vi "flame.vi"() -> ()   [LabVIEW 2017]
panel:
  in  "?":bool
  out "?":u16(ring)
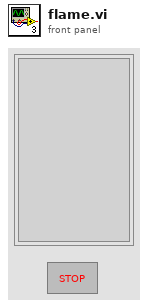
[diagram p1: front panel]
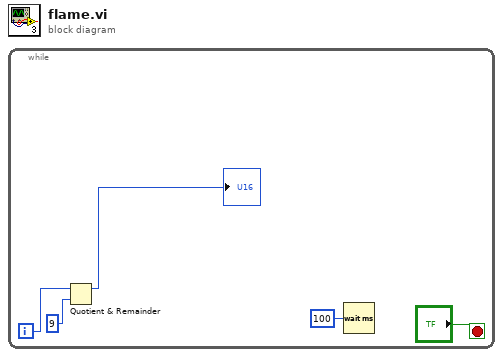
[diagram p0: block diagram]
diagram:
  n1 = while {
    i -> [w3]
    stop <- "?" stop-if-true
    n2 = Quotient & Remainder(x=w3, y=9) -> (x-y*floor(x/y)=→"?":i32)  [unwired: 1 out]
    n3 = Wait (ms)(milliseconds to wait=u32 100) -> ()  [unwired: 1 out]
  }
